vi "HW Global.vi"(6 "Clamp (Rake)":T5, 7 "HW State":T6, 8 "error in (no error)":errorcluster, 9 "servo duty cycle":dbl=0.5 format="%_6g", 10 "LED on?":bool, 11 "Hardware Info":T1={"LED Channel"="MyDigitalOutTask", "Force Sensor Channel"="Dev2/ai7", "Servo Channel"="MyPulseOutputTask", "Camera Selector"="cam5", "Camera Freq"=30.0, "FS Freq"=30.0, "Servo Freq"=30.0, "Color Pane"=0} {"Color Pane" items=["Blue", "Red", "Green", "Saturation", "Value", "Intensity", "Luminance", "Hue", ""]}) -> (0 "error out":errorcluster, 1 "Camera Data":T4, 2 "FS Data":dbl, 3 "Hardware Info out":T1={"LED Channel"="MyDigitalOutTask", "Force Sensor Channel"="Dev2/ai7", "Servo Channel"="MyPulseOutputTask", "Camera Selector"="cam5", "Camera Freq"=30.0, "FS Freq"=30.0, "Servo Freq"=30.0, "Color Pane"=0} {"Color Pane" items=["Blue", "Red", "Green", "Saturation", "Value", "Intensity", "Luminance", "Hue", ""]})   [LabVIEW 2020]
doc: "Use this template to build a VI to use as a subVI."
uses:
  Controls/HW States.ctl
  Controls/HWchannels.ctl
  <vilib>/userDefined/High Color/IMAQdx.ctl
  <vilib>/vision/Image Controls.llb/IMAQ Image.ctl
  <vilib>/DAQmx/write.llb/DAQmx Write (Digital Bool 1Line 1Point).vi
  <vilib>/DAQmx/write.llb/DAQmx Write (Counter Frequency 1Chan 1Samp).vi
  <vilib>/DAQmx/read.llb/DAQmx Read (Analog 1D DBL 1Chan NSamp).vi
  <vilib>/DAQmx/miscellaneous.llb/DAQmx Fill In Error Info.vi
  <vilib>/vision/driver/NI_Vision_Acquisition_Software.lvlib
  <vilib>/vision/NI_Vision_Development_Module.lvlib
panel:
  out "Image Dst Out":T3
  # "Channel"
  # "Frequency (Hz)"
  # "Force Sensor:"
  # "Servo:"
  # "LED:"
  # "N/A"
  # "Camera:"
  # "Channel"
  # "Frequency (Hz)"
  # "Force Sensor:"
  # "Servo:"
  # "LED:"
  # "N/A"
  # "Camera:"
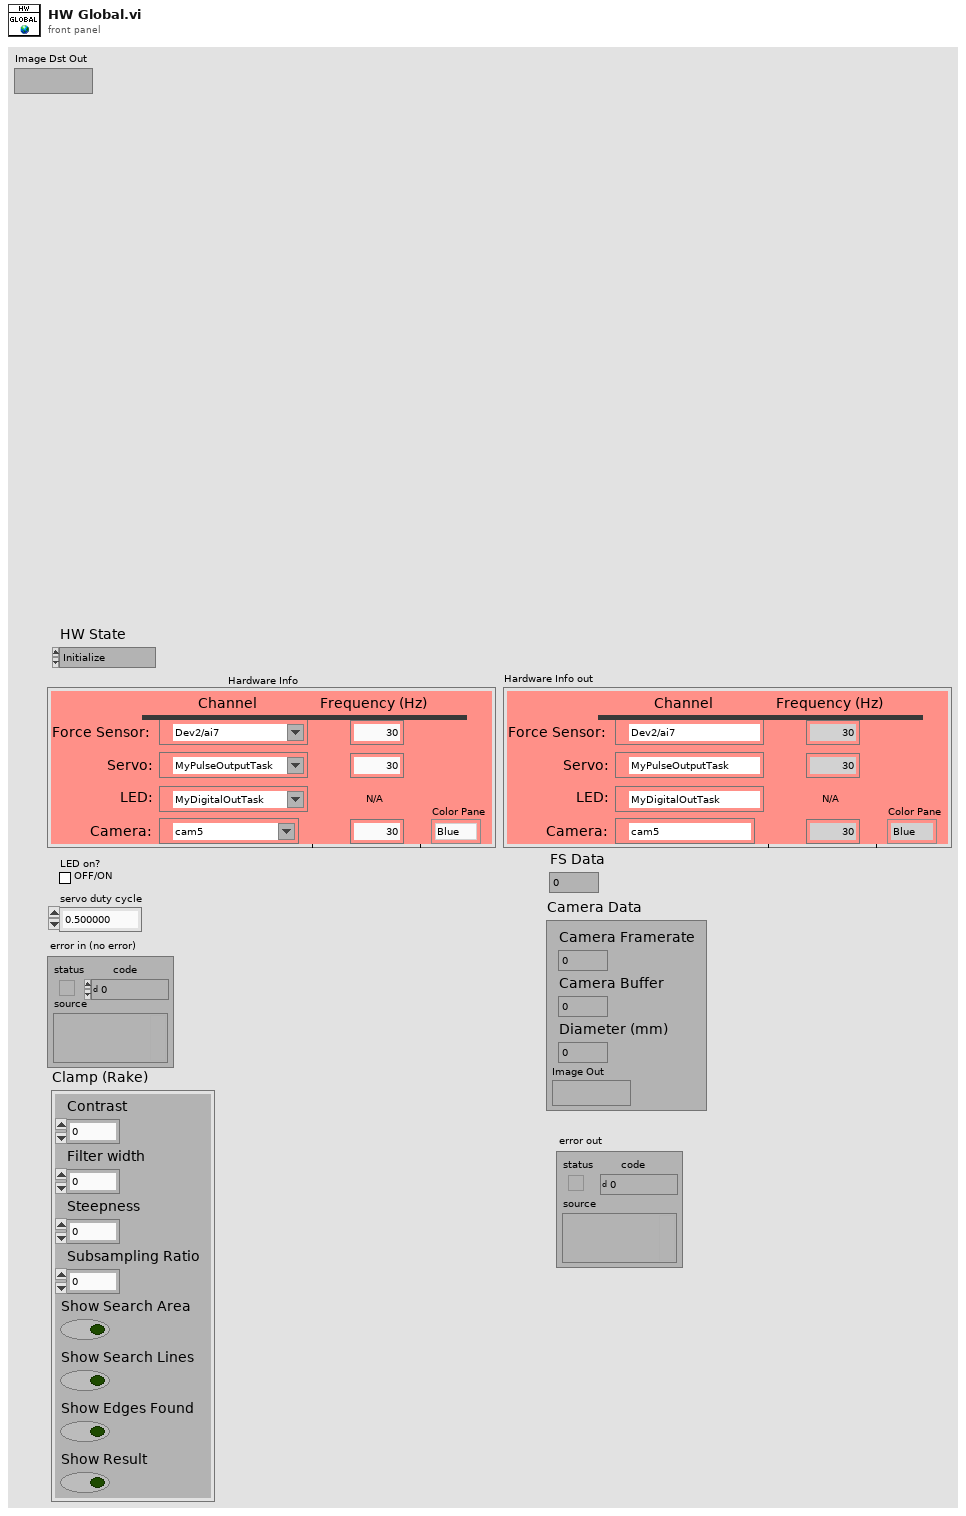
[diagram p1: front panel]
types:
  T1 = typedef "HWchannels.ctl" = cluster{"LED Channel":refnum<k21>, "Force Sensor Channel":tag, "Servo Channel":refnum<k21>, "Camera Selector":T2, "Camera Freq":dbl, "FS Freq":dbl, "Servo Freq":dbl, "Color Pane":i32}
  T2 = typedef "IMAQdx.ctl" = refnum<k21>
  T3 = typedef "IMAQ Image.ctl" = refnum<image>
  T4 = cluster{"Camera Framerate":dbl, "Camera Buffer":u32, "Diameter (mm)":dbl, "Image Out":T3}
  T5 = cluster{"Contrast":i32, "Filter width":i32, "Steepness":i32, "Subsampling Ratio":u32, "Show Search Area":bool, "Show Search Lines":bool, "Show Edges Found":bool, "Show Result":bool}
  T6 = typedef "HW States.ctl" = enum16{"Initialize", "Input LED", "Input PWM", "Acquire Voltage", "Acquire Image", "Stop"}
  T7 = cluster{"FS Task":refnum<k21>, "Servo Task":refnum<k21>, "LED Task":refnum<k21>, "Camera Session":T2, "Settings (Clamp (Rake))":cluster{"Contrast":i32, "Filter width":i32, "Steepness":i32, "Subsampling Ratio":u32, "Show Search Area":bool, "Show Search Lines":bool, "Show Edges Found":bool, "Show Result":bool}}
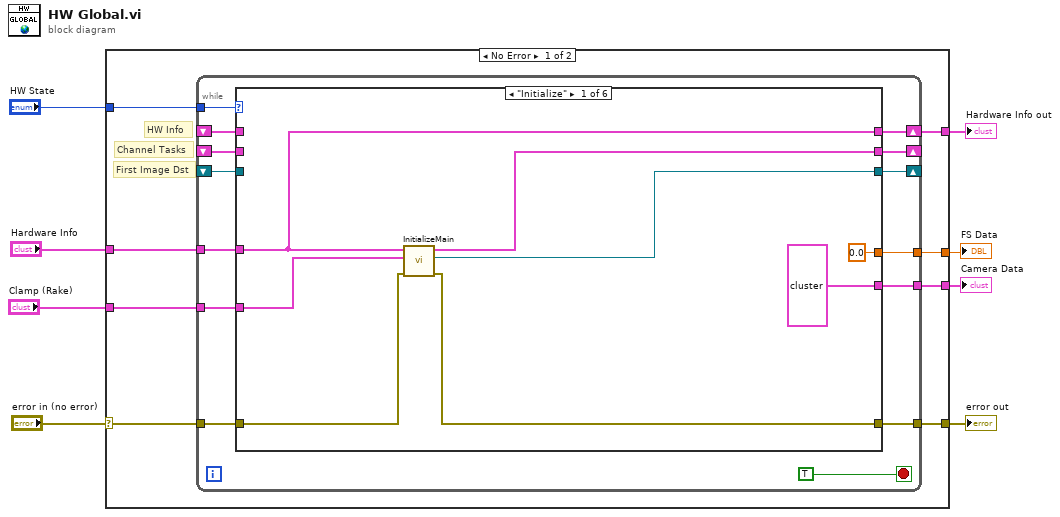
[diagram p0: block diagram]
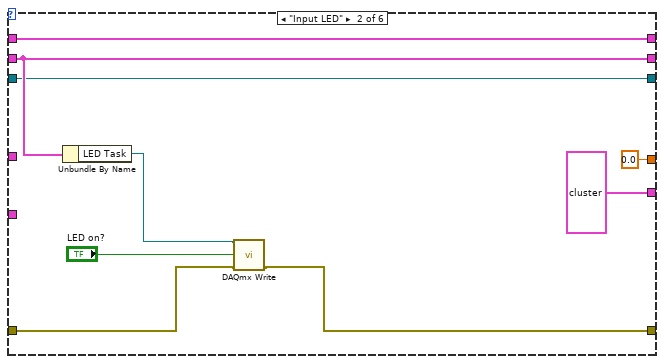
[diagram p2: hidden frame]
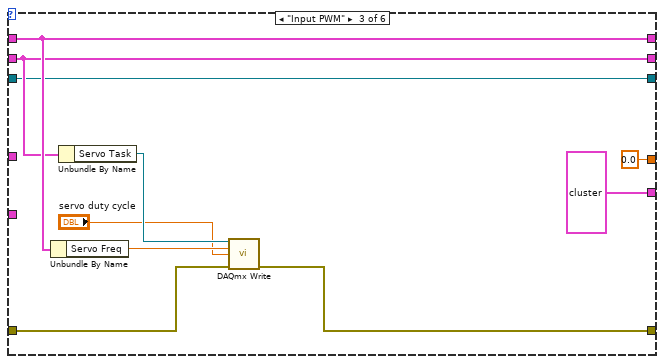
[diagram p3: hidden frame]
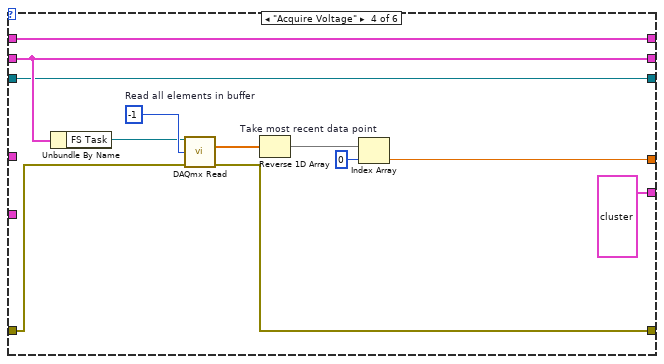
[diagram p4: hidden frame]
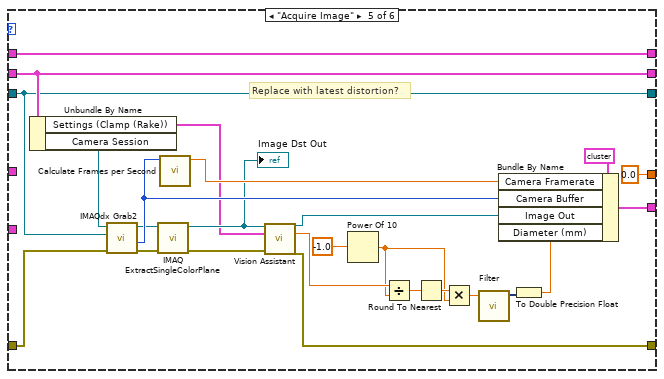
[diagram p5: hidden frame]
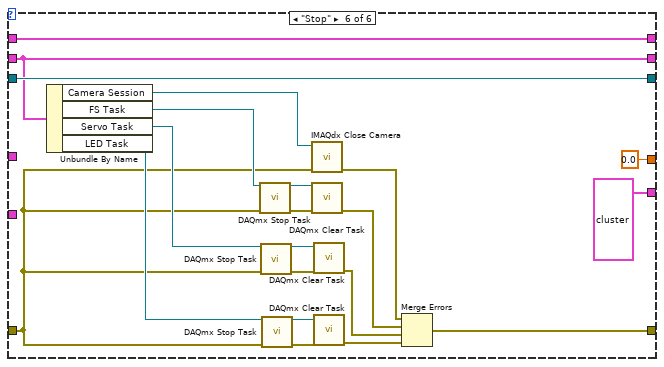
[diagram p6: hidden frame]
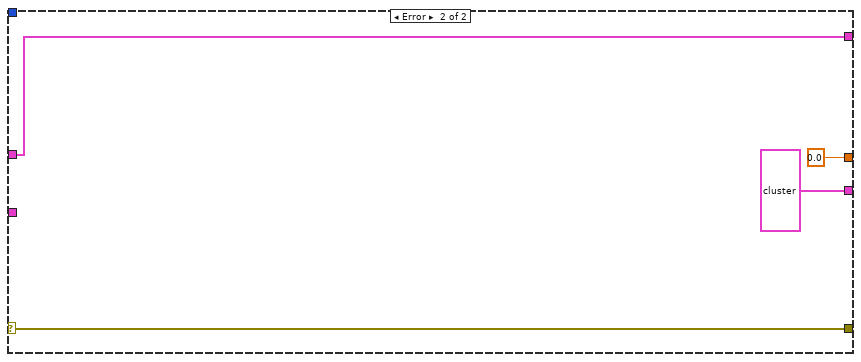
[diagram p7: hidden frame]
diagram:
  n1 = case shown="No Error" "error in (no error)" {
    selector: "error in (no error)" -> [w15 w119]
    tunnel: [w14 w119] -> w7
    tunnel: "HW State" -> [w16 _]
    tunnel: [w13 0.0 ("Waveform")] -> w5
    tunnel: "Clamp (Rake)" -> [w12 _]
    tunnel: "Hardware Info" -> [w11 w116]
    tunnel: [w10 T4 {"Camera Framerate"=0.0, "Camera Buffer"=0, "Diameter (mm)"=0.0, "Image Out"=refnum} ("input cluster")] -> w2
    tunnel: [w9 w116] -> w1
    frame No Error {
      # "First Image Dst"
      # "HW Info"
      # "Channel Tasks"
      n2 = while {
        tunnel: w16 -> [w29]
        shift-right: [w28] -> _
        shift-left: _ -> [w25]
        tunnel: w15 -> [w27]
        tunnel: [w26] -> w14
        tunnel: [w24] -> w13
        shift-right: [w23] -> w9
        shift-left: _ -> [w22]
        tunnel: w12 -> [w21]
        tunnel: w11 -> [w20]
        shift-right: [w19] -> _
        shift-left: _ -> [w18]
        tunnel: [w17] -> w10
        stop <- TRUE stop-if-true
        n3 = case shown="\"Initialize\"" w29 {
          tunnel: [w38 w46 w53 w61 w79 w99] -> w28
          tunnel: w27 -> [w37 w41 w55 w64 w76 w96]
          tunnel: [w36 w40 w49 w63 w75 w104] -> w26
          tunnel: w25 -> [_ w46 w53 w61 w79 w99]
          tunnel: [0.0 ("Waveform") 0.0 ("Waveform") 0.0 ("Waveform") w62 0.0 ("Waveform") 0.0 ("Waveform")] -> w24
          tunnel: [w34 w47 w54 w59 w94 w98] -> w23
          tunnel: w22 -> [_ w47 w54 w59 w94 w98]
          tunnel: w21 -> [w35 _ _ _ _ _]
          tunnel: w20 -> [w34 _ _ _ _ _]
          tunnel: [w33 w45 w52 w60 w70 w100] -> w19
          tunnel: w18 -> [_ w45 w52 w60 w70 w100]
          tunnel: [T4 {"Camera Framerate"=0.0, "Camera Buffer"=0, "Diameter (mm)"=0.0, "Image Out"=refnum} ("input cluster") T4 {"Camera Framerate"=0.0, "Camera Buffer"=0, "Diameter (mm)"=0.0, "Image Out"=refnum} ("input cluster") T4 {"Camera Framerate"=0.0, "Camera Buffer"=0, "Diameter (mm)"=0.0, "Image Out"=refnum} ("input cluster") T4 {"Camera Framerate"=0.0, "Camera Buffer"=0, "Diameter (mm)"=0.0, "Image Out"=refnum} ("input cluster") w74 T4 {"Camera Framerate"=0.0, "Camera Buffer"=0, "Diameter (mm)"=0.0, "Image Out"=refnum} ("input cluster")] -> w17
          frame "Initialize" {
            n4 = call "InitializeMain.vi"("error in"=w37, "Settings (Clamp (Rake))"=w35, "Hardware Info"=w34) -> ("error out"=w36:errorcluster, "New Image"=w33:T3, "Task Output"=w38:T7)  [unwired: 6 in]
          }
          frame "Input LED" {
            n5 = Unbundle By Name(w46) -> ("LED Task"=w42:refnum<k21>)
            n6 = call-poly <vilib>:"DAQmx Write.vi"("task/channels in"=w42, "data"="LED on?", "error in"=w41) -> ("error out"=w40:errorcluster)  [unwired: 10 in, 2 out]
          }
          frame "Input PWM" {
            n7 = Unbundle By Name(w54) -> ("Servo Freq"=w56:dbl)
            n8 = Unbundle By Name(w53) -> ("Servo Task"=w57:refnum<k21>)
            n9 = call-poly <vilib>:"DAQmx Write.vi"("task/channels in"=w57, "frequency"=w56, "duty cycle"="servo duty cycle", "error in"=w55) -> ("error out"=w49:errorcluster)  [unwired: 9 in, 2 out]
          }
          frame "Acquire Voltage" {
            w69 = -1  # Read all elements in buffer
            n10 = Unbundle By Name(w61) -> ("FS Task"=w65:refnum<k21>)
            n11 = call-poly <vilib>:"DAQmx Read.vi"("task/channels in"=w65, "number of samples per channel"=w69, "error in"=w64) -> ("data"=w68:dbl[], "error out"=w63:errorcluster)  [unwired: 10 in, 1 out]
            n12 = Reverse 1D Array(array=w68) -> (reversed array=w67:dbl[])
            n13 = Index Array "Take most recent data point"(array=w67, index=0) -> (element=w62:dbl)
          }
          frame "Acquire Image" {
            # "Replace with latest distortion?"
            n14 = Unbundle By Name(w79) -> ("Settings (Clamp (Rake))"=w78:T5, "Camera Session"=w77:T2)
            n15 = call <vilib>:"IMAQdx Grab2.vi"("error in"=w76, "Image In"=w70, "Session In"=w77) -> ("error out"=w83:errorcluster, "Buffer Number Out"=w93:u32, "Image Out"=w85:T3)  [unwired: 5 in, 1 out]
            n16 = call "IMAQ ExtractSingleColorPlane"("error in (no error)"=w83, "Image Src"=w85) -> ("error out"=w82:errorcluster, "Image Dst Out"=w84:T3)  [unwired: 8 in]
            "Image Dst Out" <- w84
            n17 = call <vilib>:"Calculate Frames per Second.vi"("Buffer Number"=w93) -> ("Acquired Frames/s"=w92:dbl)  [unwired: 8 in, 2 out]
            n18 = call "Vision Assistant"("Image In"=w84, "Settings (Clamp (Rake) 1)"=w78, "error in"=w82) -> ("Image Out"=w72:T3, "Distance (calibrated) (Clamp (Rake) 1)"=w90:sgl, "error out"=w75:errorcluster)  [unwired: 21 in, 1 out]
            n19 = Power Of 10(x=-1.0 ("Power of ten")) -> (10^x=w87:dbl)
            n20 = Divide(x=w90, y=w87) -> (x/y=w89:dbl)
            n21 = Round To Nearest(number=w89) -> (nearest integer value=w88:dbl)
            n22 = Multiply(x=w88, y=w87) -> (x*y=w86:dbl)
            n23 = call "Filter"("Signal"=w86) -> ("Filtered Signal"=w91:dynamicdata)  [unwired: 9 in, 1 out]
            n24 = To Double Precision Float(number=w91) -> (double precision float=w73:dbl)
            n25 = Bundle By Name(cluster=T4 {"Camera Framerate"=0.0, "Camera Buffer"=0, "Diameter (mm)"=0.0, "Image Out"=refnum} ("input cluster"), "Camera Framerate"=w92, "Camera Buffer"=w93, "Image Out"=w72, "Diameter (mm)"=w73) -> (w74:T4)
          }
          frame "Stop" {
            n26 = Unbundle By Name(w99) -> ("Camera Session"=w97:T2, "FS Task"=w101:refnum<k21>, "Servo Task"=w102:refnum<k21>, "LED Task"=w103:refnum<k21>)
            n27 = call <vilib>:"DAQmx Stop Task.vi"("task/channels in"=w101, "error in"=w96) -> ("task out"=w108:refnum<k21>, "error out"=w109:errorcluster)  [unwired: 12 in]
            n28 = call <vilib>:"DAQmx Stop Task.vi"("task/channels in"=w102, "error in"=w96) -> ("task out"=w105:refnum<k21>, "error out"=w106:errorcluster)  [unwired: 12 in]
            n29 = call <vilib>:"DAQmx Stop Task.vi"("task/channels in"=w103, "error in"=w96) -> ("task out"=w107:refnum<k21>, "error out"=w110:errorcluster)  [unwired: 12 in]
            n30 = call <vilib>:"IMAQdx Close Camera.vi"("error in"=w96, "Session In"=w97) -> ("error out"=w95:errorcluster)  [unwired: 9 in]
            n31 = call <vilib>:"DAQmx Clear Task.vi"("task in"=w108, "error in"=w109) -> ("error out"=w111:errorcluster)  [unwired: 13 in]
            n32 = call <vilib>:"DAQmx Clear Task.vi"("task in"=w105, "error in"=w106) -> ("error out"=w112:errorcluster)  [unwired: 13 in]
            n33 = call <vilib>:"DAQmx Clear Task.vi"("task in"=w107, "error in"=w110) -> ("error out"=w113:errorcluster)  [unwired: 13 in]
            n34 = Merge Errors(w95, w111, w112, w113) -> (w104:errorcluster)
          }
        }
      }
    }
    frame Error {
    }
  }
  "error out" <- w7
  "FS Data" <- w5
  "Camera Data" <- w2
  "Hardware Info out" <- w1
